vi "Close.vi"(8 "error in":errorcluster, 11 "Cycler Cluster - 24 Channel.lvclass":refnum<class "Cycler Cluster - 6 Channel.lvclass">) -> (0 "error out":errorcluster)   [LabVIEW 2023, in "Cycler Cluster - 6 Channel.lvclass"]
uses:
  Cycler Cluster - 6 Channel.lvclass
  Cycler Cluster - 6 Channel.lvclass/Cycler Cluster - 6 Channel.ctl
  <vilib>/ADAS Replay HIL/AdasHilServices/AdasHilServices Fill In Error Info Ex.vi
  <vilib>/ADAS Replay HIL/AdasHilServices/AdasHilChannelServices.lvlib
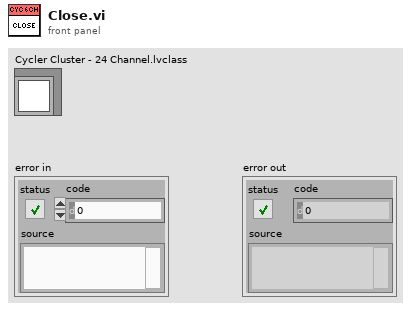
[diagram p1: front panel]
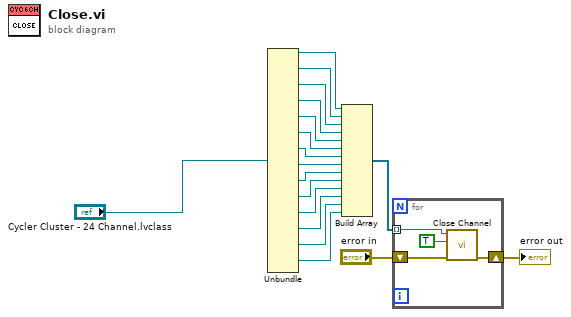
[diagram p0: block diagram]
diagram:
  n1 = Unbundle("Cycler Cluster - 24 Channel.lvclass") -> (w17:refnum<k21>, w16:refnum<k21>, w12:refnum<k21>, w11:refnum<k21>, w10:refnum<k21>, w9:refnum<k21>, w8:refnum<k21>, w7:refnum<k21>, w6:refnum<k21>, w5:refnum<k21>, w4:refnum<k21>, w3:refnum<k21>, w2:refnum<k21>, w1:refnum<k21>)  [unwired: 14 out]
  n2 = Build Array(w17, w16, w12, w11, w10, w9, w8, w7, w6, w5, w4, w3, w2, w1) -> (w15:refnum<k21>[])
  n3 = for {
    tunnel: w15 -> [w22] mode=indexing
    shift-right: [w19] -> w13
    shift-left: "error in" -> [w20]
    n4 = call <vilib>:"Close Channel.vi"("error in"=w20, "Force Destroy? (F)"=TRUE, "ADAS HIL Channel"=w22) -> ("error out"=w19:errorcluster)  [unwired: 8 in]
  }
  "error out" <- w13
